vi "resonancia.vi"() -> ()   [LabVIEW 2010]
uses:
  <vilib>/sound2/lvsound2.llb/Sound Data Format.ctl
  <vilib>/sound2/lvsound2.llb/Sampling Mode.ctl
  <vilib>/sound2/lvsound2.llb/Sound Output Write (DBL Single).vi
  <vilib>/Utility/file.llb/Write To Spreadsheet File (DBL).vi
  <vilib>/sound2/lvsound2.llb/Sound Input Read (DBL).vi
  <vilib>/measure/matone.llb/Extract Single Tone Information N Chan.vi
  <vilib>/measure/madcrms.llb/Basic Averaged DC-RMS for N Chan.vi
  <vilib>/measure/NI_MAPro.lvlib
panel:
  out "detected frequencies":dbl[](array[numeric]) format="%.2p"
  out "detected amplitudes":dbl[](graph)
  out "RMS values":dbl[](graph)
  out "data":waveform(dbl)[](graph)
  in  "number of samples/ch":i32=100000
  out "x/y":dbl
  out "Frecuencia":i32
  in  "Sound Format":T1={"sample rate (S/s)"=44100.0, "number of channels"=2, "bits per sample"=16}
  in  "tiempo (ms)":dbl=20000.0
  in  "Input Device ID":u32
  in  "Output Device ID":u32
  in  "stop":bool
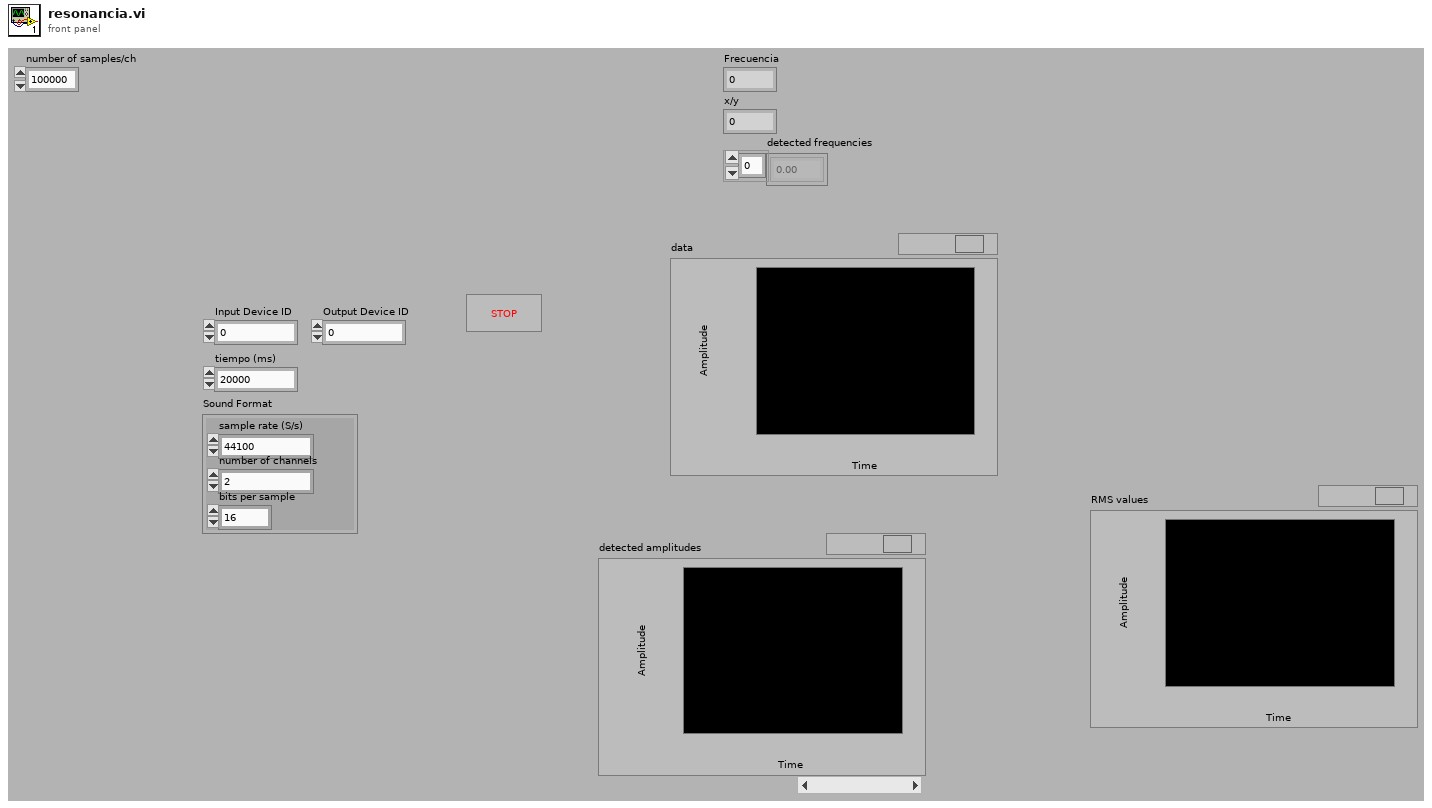
[diagram p1: front panel]
types:
  T1 = typedef "Sound Data Format.ctl" = cluster{"sample rate (S/s)":dbl, "number of channels":i32, "bits per sample":i32}
  T2 = typedef "Sampling Mode.ctl" = i32
  T3 = typedef "Sound Output Task ID.ctl" = u32
  T4 = typedef "Sound Input Task ID.ctl" = u32
  T5 = enum32{"none", "input signal", "detected signal", "residual signal"}
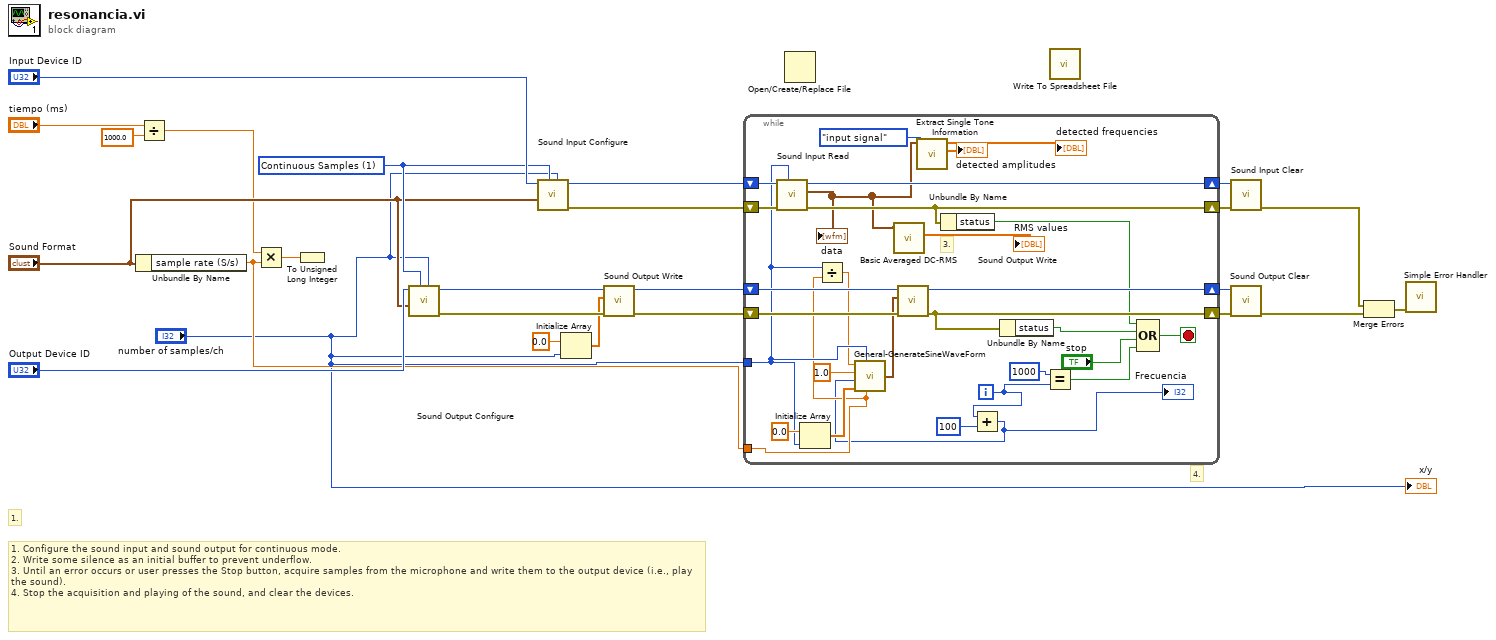
[diagram p0: block diagram]
diagram:
  w15 = T2 1 items=["Finite Samples", "Continuous Samples"] ("sample mode")
  # "4."
  # "1."
  # "1. Configure the sound input and sound output for continuous mode.\n2. Write some silence as an initial buffer to prevent underflow.\n3. Until an error occurs or user presses the Stop button, acquire samples from the microphone and write them to the output device (i.e., play the sound).\n4. Stop the acquisition and playing of the sound, and clear the devices."
  n1 = Unbundle By Name("Sound Format") -> ("sample rate (S/s)"=w4:dbl)
  n2 = Divide(x="tiempo (ms)", y=1000.0) -> (x/y=w2:dbl)
  n3 = Multiply(x=w2, y=w4) -> (x*y=w3:dbl)
  n4 = To Unsigned Long Integer(number=w3) -> ()  [unwired: 1 out]
  n5 = call <vilib>:"Sound Output Configure.vi"("number of samples/ch"="number of samples/ch", "sample mode"=w15, "sound format"="Sound Format", "device ID"="Output Device ID") -> ("error out"=w13:errorcluster, "task ID"=w14:T3)  [unwired: 6 in]
  n6 = call <vilib>:"Sound Input Configure.vi"("number of samples/ch"="number of samples/ch", "sample mode"=w15, "sound format"="Sound Format", "device ID"="Input Device ID") -> ("error out"=w17:errorcluster, "task ID"=w16:T4)  [unwired: 6 in]
  n7 = Initialize Array(0.0 ("element"), "number of samples/ch") -> (w8:dbl[])
  n8 = call-poly <vilib>:"Sound Output Write.vi"("error in (no error)"=w13, "data"=w8, "task ID"=w14) -> ("error out"=w12:errorcluster, "task ID out"=w11:T3)  [unwired: 7 in]
  n9 = while {
    shift-right: [w47] -> w24
    shift-left: w12 -> [w49]
    shift-right: [w48] -> w25
    shift-left: w17 -> [w54]
    shift-right: [w51] -> w23
    shift-left: w11 -> [w53]
    shift-right: [w50] -> w20
    shift-left: w16 -> [w52]
    tunnel: w4 -> [w35]
    tunnel: "number of samples/ch" -> [w36]
    i -> [w32]
    stop <- w43 stop-if-true
    # "3."
    n10 = call-poly <vilib>:"Sound Input Read.vi"("number of samples/ch"=w36, "error in (no error)"=w54, "task ID"=w52) -> ("error out"=w48:errorcluster, "data"=w29:waveform(dbl)[], "task ID out"=w50:T4)  [unwired: 6 in]
    "data" <- w29
    n11 = Initialize Array(0.0 ("element"), w36) -> (w41:dbl[])
    n12 = Divide(x=w36, y=w35) -> (x/y=w34:dbl)
    n13 = call-poly <vilib>:"Basic Averaged DC-RMS.vi"("signals in"=w29) -> ("RMS values"=→"RMS values":dbl[])  [unwired: 7 in, 3 out]
    n14 = call-poly <vilib>:"Extract Single Tone Information.vi"("export mode"=T5."input signal", "time signals in"=w29) -> ("detected amplitudes"=→"detected amplitudes":dbl[], "detected frequencies"=→"detected frequencies":dbl[])  [unwired: 4 in, 4 out]
    n15 = Unbundle By Name(w48) -> ("status"=w44:bool)
    n16 = Add(x=w32, y=100) -> (x+y=w31:i32)
    "Frecuencia" <- w31
    n17 = call "General-GenerateSineWaveForm.vi"("tiempo (s)"=w34, "#samples"=w36, "Amplitud"=1.0, "frecuencia"=w31, "Fs (S/s)"=w35, "df"=w41) -> ("Waveform"=w37:waveform(dbl))  [unwired: 2 in]
    n18 = call-poly <vilib>:"Sound Output Write.vi"("error in (no error)"=w49, "data"=w37, "task ID"=w53) -> ("error out"=w47:errorcluster, "task ID out"=w51:T3)  [unwired: 7 in]
    n19 = Unbundle By Name(w47) -> ("status"=w45:bool)
    n20 = Equal?(x=1000, y=w32) -> (x = y?=w39:bool)
    n21 = Compound Arithmetic op=OR(w44, w45, "stop", w39) -> (w43:bool)
  }
  n22 = Open/Create/Replace File() -> ()  [unwired: 6 in, 3 out]
  n23 = call-poly <vilib>:"Write To Spreadsheet File.vi"() -> ()  [unwired: 8 in, 1 out]
  n24 = call <vilib>:"Sound Input Clear.vi"("error in (no error)"=w25, "task ID"=w20) -> ("error out"=w18:errorcluster)  [unwired: 9 in]
  n25 = call <vilib>:"Sound Output Clear.vi"("error in (no error)"=w24, "task ID"=w23) -> ("error out"=w19:errorcluster)  [unwired: 9 in]
  n26 = Merge Errors(w18, w19) -> (w10:errorcluster)
  n27 = call <vilib>:"Simple Error Handler.vi"("error in (no error)"=w10) -> ()  [unwired: 4 in, 5 out]
  "x/y" <- "number of samples/ch"
